vi "Invert.vi"(0 "image in":refnum<class "MSC Image.lvclass">, 5 "error in (no error)":errorcluster) -> (14 "image out":refnum<class "MSC Image.lvclass">, 19 "error out":errorcluster)   [LabVIEW 2014, in "MSC Image.lvclass"]
doc: "Inverts the image."
uses:
  MSC Image.lvclass
  MSC Image.lvclass/MSC Image.ctl
  Dependencies/x86/MSC I Process32.dll
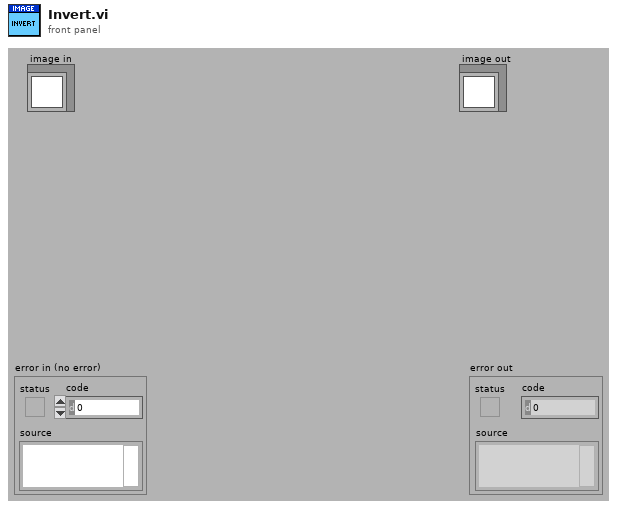
[diagram p1: front panel]
types:
  T1 = typedef "Image.ctl" = cluster{"Pointer":u64, "Size":T2, "Image Type":T3, "Time Stamp":timestamp, "Variant":variant}
  T2 = typedef "Size.ctl" = cluster{"Cols":i32, "Rows":i32}
  T3 = typedef "Image Type.ctl" = i32
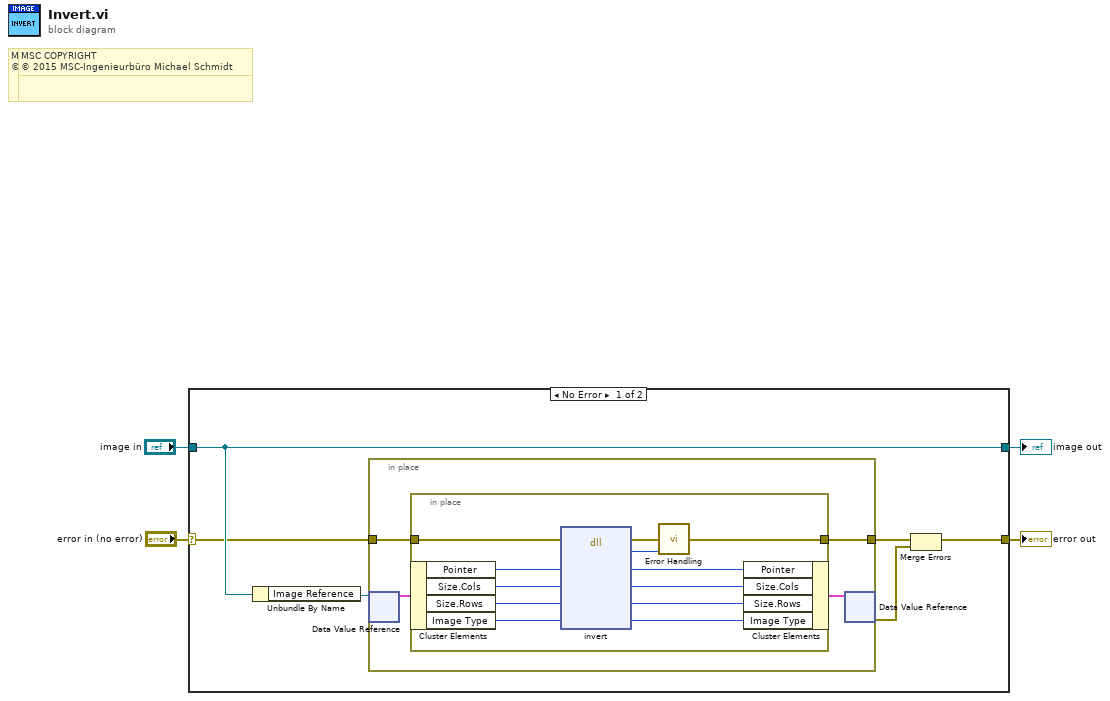
[diagram p0: block diagram]
diagram:
  # "MSC COPYRIGHT\n© 2016 MSC-Ingenieurbüro Michael Schmidt"
  # "MSC COPYRIGHT\n© 2016 MSC-Ingenieurbüro Michael Schmidt"
  # "MSC COPYRIGHT\n© 2015 MSC-Ingenieurbüro Michael Schmidt"
  # "MSC COPYRIGHT\n© 2015 MSC-Ingenieurbüro Michael Schmidt"
  n1 = case shown="No Error" "error in (no error)" {
    selector: "error in (no error)" -> [w6 w28]
    tunnel: [w5 w28] -> w3
    tunnel: [w10 w27] -> w1
    tunnel: "image in" -> [w10 w27]
    frame No Error {
      n2 = Unbundle By Name(w10) -> ("Image Reference"=w9:refnum<data-value>)
      n3 = in-place {
        in-place-border: w6 -> [w12]
        in-place-border: [w11] -> w8
        n4 = in-place-dvr #1(w9) -> (w13:T1)  [unwired: 1 out]
        n5 = in-place {
          in-place-border: w12 -> [w25]
          in-place-border: [w26] -> w11
          n6 = in-place-cluster #2(w13) -> ("Pointer"=w22:u64, "Size.Cols"=w21:i32, "Size.Rows"=w20:i32, "Image Type"=w19:T3)
          n7 = dll-call lib="C:/Users/MSC/LabVIEW Projekte/LV 2014/MSC I-Process/user.lib/MSC-I Process/Dependencies/x86/MSC I Process*.dll" fn="invert"(error in=w25, "pointer"=w22, "cols"=w21, "rows"=w20, "type"=w19) -> (error out=w24:errorcluster, "error"=w23:i32, "pointer"=w15:u64, "cols"=w16:i32, "rows"=w17:i32, "type"=w18:i32)  [unwired: 2 in, 1 out]
          n8 = call "Error Handling.vi"("error in (no error)"=w24, "return type"=w23) -> ("error out"=w26:errorcluster)  [unwired: 12 in, 1 out]
          n9 = in-place-cluster #2("Pointer"=w15, "Size.Cols"=w16, "Size.Rows"=w17, "Image Type"=w18) -> (w14:T1)
        }
        n10 = in-place-dvr #1(w14) -> (w7:errorcluster)  [unwired: 1 out]
      }
      n11 = Merge Errors(w8, w7) -> (w5:errorcluster)
    }
    frame Error {
    }
  }
  "error out" <- w3
  "image out" <- w1
